vi "Shared Var Loop.vi"(0 "reference in":refnum<class "Stand.lvclass">, 11 "error in (no error)":errorcluster) -> (4 "reference in 2":refnum<class "Stand.lvclass">, 15 "error out":errorcluster)   [LabVIEW 2019, in "Stand.lvclass"]
uses:
  Stand.lvclass
  TypeDef/NVM Data.ctl
  modbus engine custom/MB_ENGINE_class/Engine Alarms.ctl
  modbus engine custom/MB_ENGINE_class/Engine State.ctl
  TypeDef/StateValveModbus.ctl
  modbus engine custom/MB_ENGINE_class/Settings.ctl
  Stand.lvclass/Stand.ctl
  ValveModbus_class/ValveModbus.lvclass/ValveModbus.ctl
  Engine_1DI_2DO_class/Engine_1DI_2DO.lvclass/Engine_1DI_2DO.ctl
  Sig_DA_class/Sig_DA.lvclass/Sig_DA.ctl
  TypeDef/DA_Data.ctl
  TypeDef/bool_data.ctl
  TypeDef/State HI_PERESS_TEST.ctl
  TypeDef/State.ctl
  Sig_AO_class/Sig_AO.lvclass/Sig_AO.ctl
  Sig_DO_Simple_class/Sig_DO_Simple.lvclass/Sig_DO_Simple.ctl
  Sig_DI_Simple_class/Sig_DI_Simple.lvclass/Sig_DI_Simple.ctl
  Sig_AI_class/Sig_AI.lvclass/Sig_AI.ctl
  AnalogComparator_class/AnalogComparator.lvclass/AnalogComparator.ctl
  TypeDef/AI_Data_Array.ctl
  TypeDef/AI_Data.ctl
  TypeDef/PumpData.ctl
  TypeDef/StatePump.ctl
  AnalogComparator_class/GetStatus.vi
  AnalogComparator_class/GetTh.vi
  modbus engine custom/MB_ENGINE_class/MB_ENGINE.lvclass
  Sig_AI_class/Sig_AI.lvclass
  Sig_DI_Simple_class/Sig_DI_Simple.lvclass
  Sig_DO_Simple_class/Sig_DO_Simple.lvclass
  Sig_AO_class/Sig_AO.lvclass
  Engine_1DI_2DO_class/Engine_1DI_2DO.lvclass
  Sig_DA_class/Sig_DA.lvclass
  ValveModbus_class/ValveModbus.lvclass
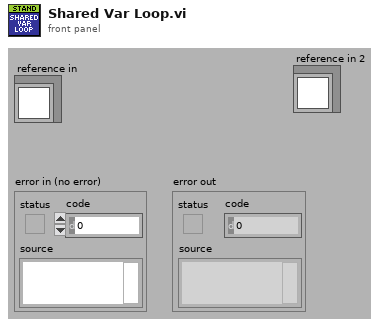
[diagram p1: front panel]
types:
  T1 = typedef "NVM Data.ctl" = cluster{"Alarms":T2, "Engine State":T3, "RAW Possition":i32, "StateValveModbus":T4, "Angele":dbl, "Step":i32, "Encoder":i32, "Kinematic":T5}
  T2 = typedef "MB_ENGINE.lvclass/Engine Alarms.ctl" = cluster{"OL":bool, "TF":bool, "STL":bool, "OCP":bool, "CPUV":bool, "UVLO":bool, "SPI_ERROR":bool, "Fault":bool, "OL 2":bool, "TF 2":bool, "STL 2":bool, "OCP 2":bool, "CPUV 2":bool, "UVLO 2":bool, "reserved":bool, "InitDone":bool}
  T3 = typedef "MB_ENGINE.lvclass/Engine State.ctl" = u16
  T4 = typedef "StateValveModbus.ctl" = enum16{"IDLE", "OPEN", "CLOSE", "OPENING", "CLOSING", "STOP"}
  T5 = typedef "MB_ENGINE.lvclass/Settings.ctl" = cluster{"ACC Steps Per Sec^2":u16, "DEC Steps Per Sec^2":u16, "Min Velosity Step Per Sec":u16, "Max Velosity Step Per Sec":u16, "MicroStep":u16}
  T6 = typedef "State.ctl" = enum16{"INIT", "IDLE", "CHANNEL_TESTING", "OIL_FILLING", "PREPARE_TO_HI_PRESS", "HI_PRESSURE", "ALARM", "HI PRESSURE TEST"}
  T7 = typedef "State HI_PERESS_TEST.ctl" = enum16{"NOT READY", "READY TO SUPPLY AIR", "PREPARE TO HI PRESS", "READY FOR HI PRESS", "CHECK DIRECTION", "INCREASING PRESSURE", "HOLDING", "PRESSURE RELEASE", "SOFT PRESSURE RELIEF", "ALARM"}
  T8 = typedef "StatePump.ctl" = enum16{"Off", "TupningOn", "On", "TurningOff"}
  T9 = typedef "AI_Data.ctl" = cluster{"Raw":dbl, "Scaled":dbl, "OutOfRangeMax":bool, "OutOfRangeMin":bool, "HIHI":bool, "HI":bool, "LO":bool, "LOLO":bool, "OutOfRangeMax_val":dbl, "OutOfRangeMin_val":dbl, "HIHI_val":dbl, "HI_val":dbl, "LO_val":dbl, "LOLO_val":dbl}
  T10 = typedef "bool_data.ctl" = cluster{"CURR":bool, "RAW_PREV":bool, "millisecond timer value":u32}
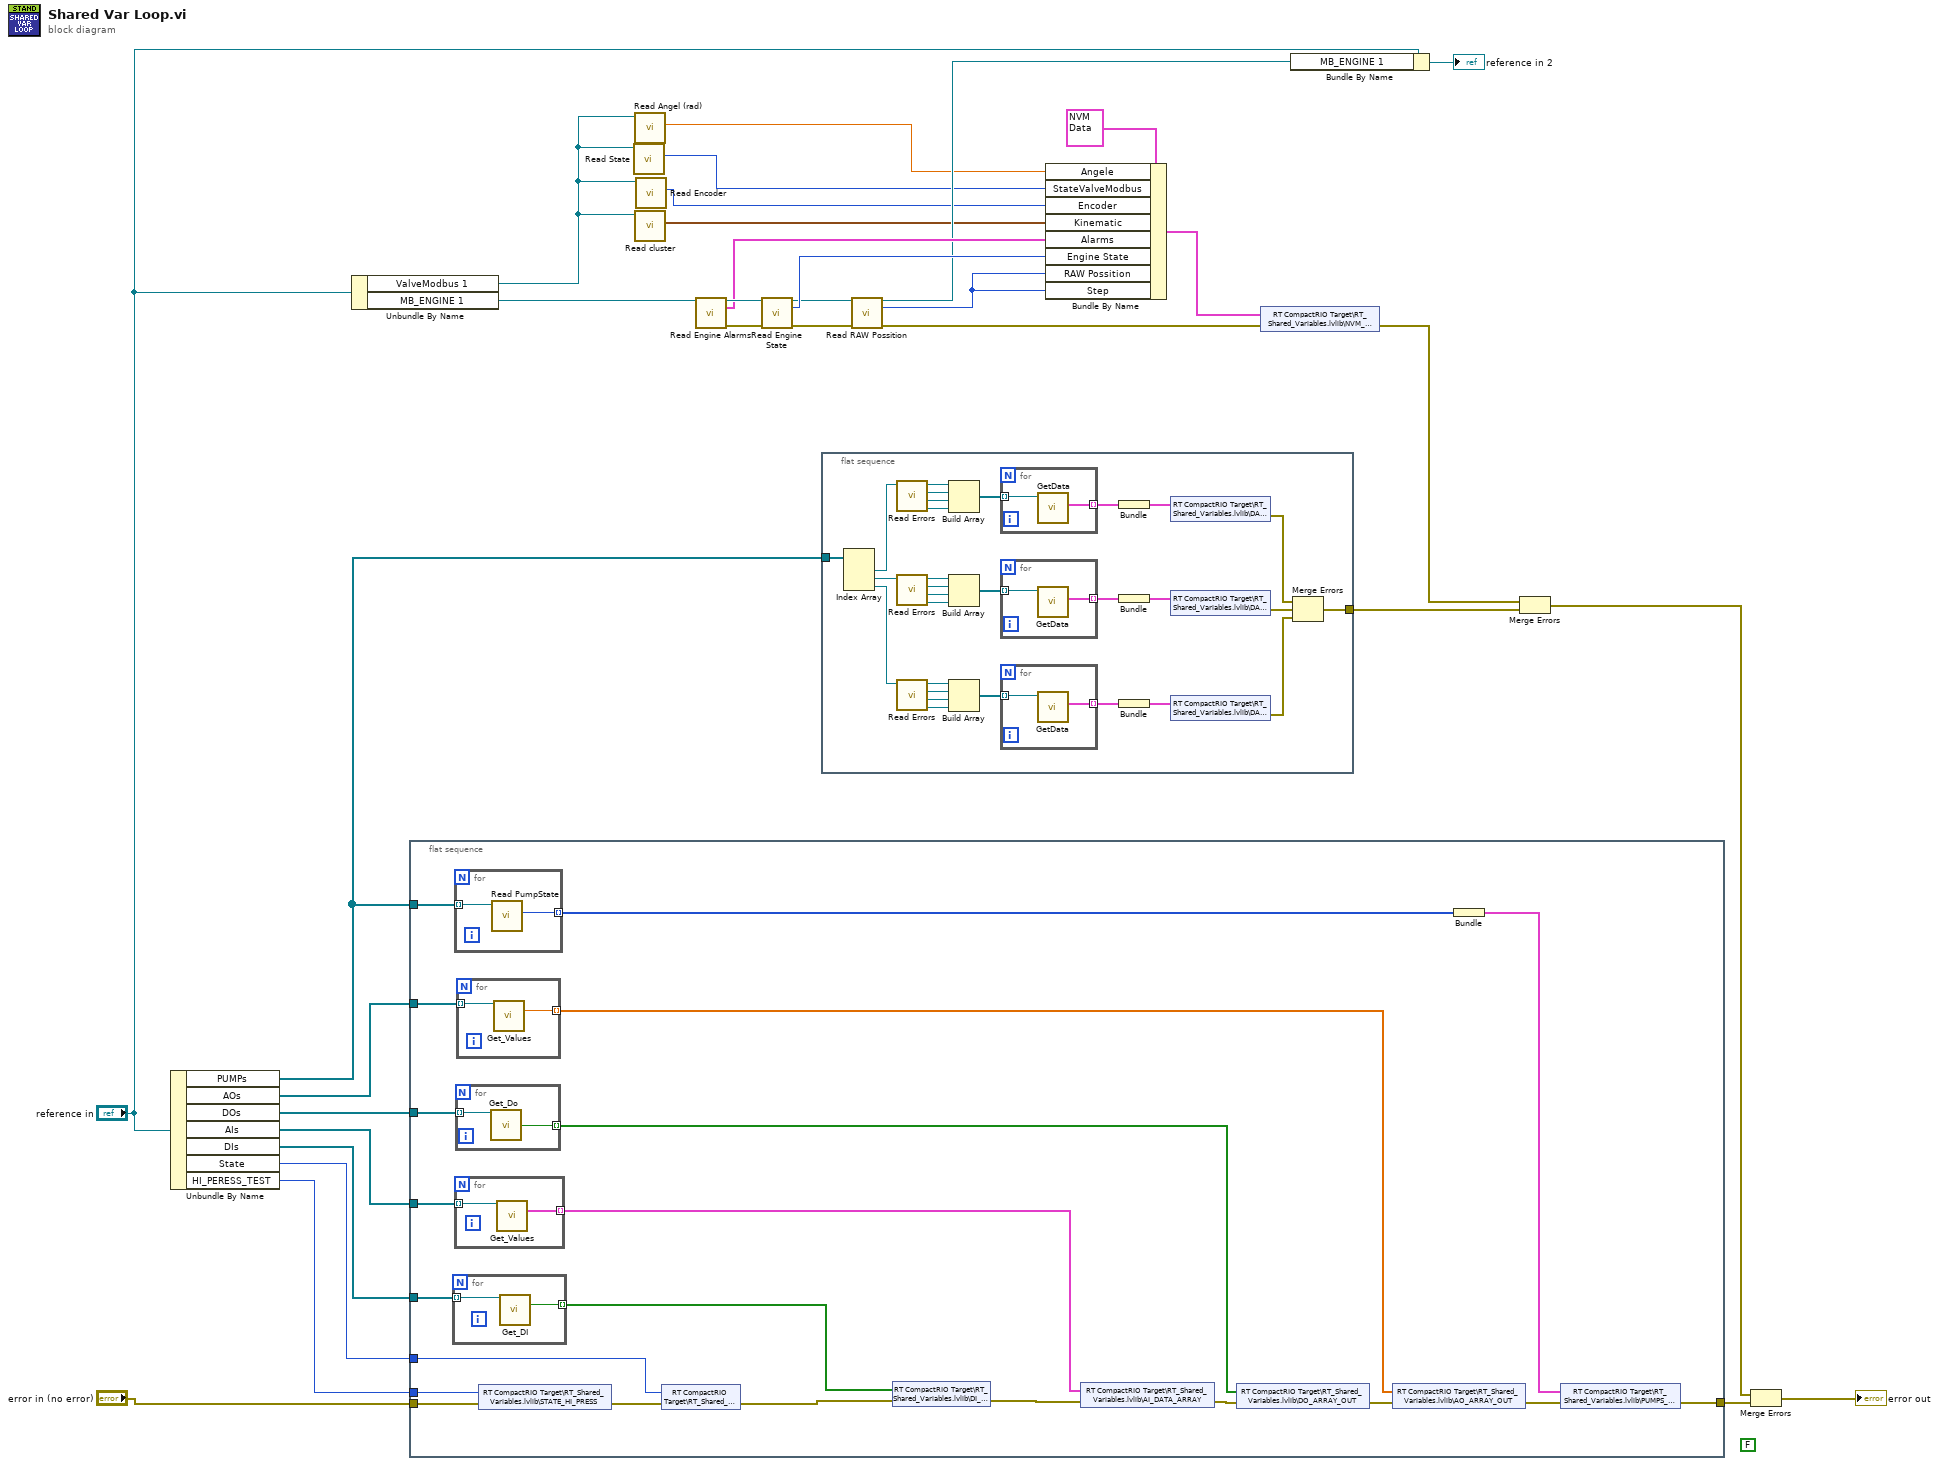
[diagram p0: block diagram]
diagram:
  (unwired) FALSE
  n1 = Unbundle By Name("reference in") -> ("PUMPs"=w27:refnum<class "Engine_1DI_2DO.lvclass">[], "AOs"=w28:refnum<class "Sig_AO.lvclass">[], "DOs"=w29:refnum<class "Sig_DO_Simple.lvclass">[], "AIs"=w31:refnum<class "Sig_AI.lvclass">[], "DIs"=w30:refnum<class "Sig_DI_Simple.lvclass">[], "State"=w23:T6, "HI_PERESS_TEST"=w1:T7)
  n2 = Unbundle By Name("reference in") -> ("ValveModbus 1"=w6:refnum<class "ValveModbus.lvclass">, "MB_ENGINE 1"=w14:refnum<class "MB_ENGINE.lvclass">)
  n3 = flat-sequence {
    tunnel: w31 -> [w53]
    tunnel: w30 -> [w51]
    tunnel: w29 -> [w49]
    tunnel: w28 -> [w47]
    tunnel: w27 -> [w41]
    tunnel: [w40] -> w26
    tunnel: "error in (no error)" -> [w34]
    tunnel: w23 -> [w39]
    tunnel: w1 -> [w35]
    frame #0 {
      n4 = for {
        tunnel: w51 -> [w61] mode=indexing
        tunnel: [w60] -> w38 mode=indexing
        n5 = call "Get_DI.vi"("reference in"=w61) -> ("DI"=w60:bool)  [unwired: 14 in]
      }
      n6 = for {
        tunnel: w41 -> [w55] mode=indexing
        tunnel: [w54] -> w43 mode=indexing
        n7 = call "Read PumpState.vi"("Pump_1AI_1DO_2DI in"=w55) -> ("PumpState"=w54:T8)  [unwired: 10 in]
      }
      n8 = for {
        tunnel: w53 -> [w63] mode=indexing
        tunnel: [w62] -> w52 mode=indexing
        n9 = call "Get_Values.vi"("reference in"=w63) -> ("Data"=w62:T9)  [unwired: 13 in, 1 out]
      }
      n10 = for {
        tunnel: w49 -> [w59] mode=indexing
        tunnel: [w58] -> w50 mode=indexing
        n11 = call "Get_Do.vi"("reference in"=w59) -> ("DO"=w58:bool)  [unwired: 14 in]
      }
      n12 = for {
        tunnel: w47 -> [w57] mode=indexing
        tunnel: [w56] -> w45 mode=indexing
        n13 = call "Get_Values.vi"("reference in"=w57) -> ("AO"=w56:dbl)  [unwired: 14 in]
      }
      n14 = shared-variable "RT CompactRIO Target\\RT_Shared_Variables.lvlib\\STATE_HI_PRESS"(w35, error in=w34) -> (error out=w33:errorcluster)
      n15 = shared-variable "RT CompactRIO Target\\RT_Shared_Variables.lvlib\\STATE"(w39, error in=w33) -> (error out=w37:errorcluster)
      n16 = shared-variable "RT CompactRIO Target\\RT_Shared_Variables.lvlib\\DI_ARRAY"(w38, error in=w37) -> (error out=w36:errorcluster)
      n17 = shared-variable "RT CompactRIO Target\\RT_Shared_Variables.lvlib\\AI_DATA_ARRAY"(w52, error in=w36) -> (error out=w48:errorcluster)
      n18 = shared-variable "RT CompactRIO Target\\RT_Shared_Variables.lvlib\\DO_ARRAY_OUT"(w50, error in=w48) -> (error out=w46:errorcluster)
      n19 = shared-variable "RT CompactRIO Target\\RT_Shared_Variables.lvlib\\AO_ARRAY_OUT"(w45, error in=w46) -> (error out=w44:errorcluster)
      n20 = Bundle(w43) -> (w42:cluster{T8[]})  [unwired: 1 in]
      n21 = shared-variable "RT CompactRIO Target\\RT_Shared_Variables.lvlib\\PUMPS_DATA"(w42, error in=w44) -> (error out=w40:errorcluster)
    }
  }
  n22 = call "Read State.vi"("Pump_1AI_1DO_2DI in"=w6) -> ("StateValveModbus"=w7:T4)  [unwired: 10 in]
  n23 = call "Read Angel (rad).vi"("ValveModbus in"=w6) -> ("Angel (rad)"=w5:dbl)  [unwired: 9 in, 1 out]
  n24 = call "Read cluster.vi"("ValveModbus in"=w6) -> ("cluster"=w8:T5)  [unwired: 9 in, 1 out]
  n25 = call "Read Encoder.vi"("ValveModbus in"=w6) -> ("Encoder"=w9:i32)  [unwired: 9 in, 1 out]
  n26 = call-dynamic "Read Engine Alarms.vi"("class data in"=w14) -> ("class data out"=w20:refnum<class "MB_ENGINE.lvclass">, "Alarms"=w18:T2, "error out"=w19:errorcluster)  [unwired: 12 in]
  n27 = call-dynamic "Read Engine State.vi"("class data in"=w20, "error in (no error)"=w19) -> ("class data out"=w16:refnum<class "MB_ENGINE.lvclass">, "Engine State"=w17:T3, "error out"=w15:errorcluster)  [unwired: 11 in]
  n28 = flat-sequence {
    tunnel: w27 -> [w92]
    tunnel: [w64] -> w25
    frame #0 {
      n29 = Index Array(array=w92) -> (element #1=w87:refnum<class "Engine_1DI_2DO.lvclass">, element #2=w82:refnum<class "Engine_1DI_2DO.lvclass">, element #3=w79:refnum<class "Engine_1DI_2DO.lvclass">)  [unwired: 3 in]
      n30 = call "Read Errors.vi"("Pump_1AI_1DO_2DI in"=w87) -> ("UnOFF Error"=w88:refnum<class "Sig_DA.lvclass">, "UnON Error"=w89:refnum<class "Sig_DA.lvclass">, "OFF Error"=w90:refnum<class "Sig_DA.lvclass">, "ON Error"=w91:refnum<class "Sig_DA.lvclass">)  [unwired: 7 in]
      n31 = call "Read Errors.vi"("Pump_1AI_1DO_2DI in"=w82) -> ("UnOFF Error"=w86:refnum<class "Sig_DA.lvclass">, "UnON Error"=w85:refnum<class "Sig_DA.lvclass">, "OFF Error"=w84:refnum<class "Sig_DA.lvclass">, "ON Error"=w83:refnum<class "Sig_DA.lvclass">)  [unwired: 7 in]
      n32 = call "Read Errors.vi"("Pump_1AI_1DO_2DI in"=w79) -> ("UnOFF Error"=w80:refnum<class "Sig_DA.lvclass">, "UnON Error"=w81:refnum<class "Sig_DA.lvclass">, "OFF Error"=w77:refnum<class "Sig_DA.lvclass">, "ON Error"=w78:refnum<class "Sig_DA.lvclass">)  [unwired: 7 in]
      n33 = Build Array(w91, w90, w89, w88) -> (w76:refnum<class "Sig_DA.lvclass">[])
      n34 = Build Array(w83, w84, w85, w86) -> (w72:refnum<class "Sig_DA.lvclass">[])
      n35 = Build Array(w78, w77, w81, w80) -> (w71:refnum<class "Sig_DA.lvclass">[])
      n36 = for {
        tunnel: w76 -> [w98] mode=indexing
        tunnel: [w97] -> w74 mode=indexing
        n37 = call "GetData.vi"("Sig_DA in"=w98) -> ("data"=w97:T10)  [unwired: 10 in]
      }
      n38 = for {
        tunnel: [w96] -> w73 mode=indexing
        tunnel: w72 -> [w95] mode=indexing
        n39 = call "GetData.vi"("Sig_DA in"=w95) -> ("data"=w96:T10)  [unwired: 10 in]
      }
      n40 = for {
        tunnel: [w94] -> w70 mode=indexing
        tunnel: w71 -> [w93] mode=indexing
        n41 = call "GetData.vi"("Sig_DA in"=w93) -> ("data"=w94:T10)  [unwired: 10 in]
      }
      n42 = Bundle(w74) -> (w75:cluster{T10[]})  [unwired: 1 in]
      n43 = Bundle(w73) -> (w68:cluster{T10[]})  [unwired: 1 in]
      n44 = Bundle(w70) -> (w69:cluster{T10[]})  [unwired: 1 in]
      n45 = shared-variable "RT CompactRIO Target\\RT_Shared_Variables.lvlib\\DA_ENG_0"(w75) -> (error out=w65:errorcluster)  [unwired: 1 in]
      n46 = shared-variable "RT CompactRIO Target\\RT_Shared_Variables.lvlib\\DA_ENG_1"(w68) -> (error out=w66:errorcluster)  [unwired: 1 in]
      n47 = shared-variable "RT CompactRIO Target\\RT_Shared_Variables.lvlib\\DA_ENG_2"(w69) -> (error out=w67:errorcluster)  [unwired: 1 in]
      n48 = Merge Errors(w65, w66, w67) -> (w64:errorcluster)
    }
  }
  n49 = call-dynamic "Read RAW Possition.vi"("class data in"=w16, "error in (no error)"=w15) -> ("class data out"=w11:refnum<class "MB_ENGINE.lvclass">, "RAW Possition"=w10:i32, "error out"=w4:errorcluster)  [unwired: 11 in]
  n50 = Bundle By Name(cluster=T1 {"Alarms"={"OL"=FALSE, "TF"=FALSE, "STL"=FALSE, "OCP"=FALSE, "CPUV"=FALSE, "UVLO"=FALSE, "SPI_ERROR"=FALSE, "Fault"=FALSE, "OL 2"=FALSE, "TF 2"=FALSE, "STL 2"=FALSE, "OCP 2"=FALSE, "CPUV 2"=FALSE, "UVLO 2"=FALSE, "reserved"=TRUE, "InitDone"=TRUE}, "Engine State"=8, "RAW Possition"=124110, "StateValveModbus"=enum."IDLE", "Angele"=0.0, "Step"=0, "Encoder"=0, "Kinematic"={"ACC Steps Per Sec^2"=100, "DEC Steps Per Sec^2"=100, "Min Velosity Step Per Sec"=100, "Max Velosity Step Per Sec"=200, "MicroStep"=16}} ("NVM_DATA_1"), "Angele"=w5, "StateValveModbus"=w7, "Encoder"=w9, "Kinematic"=w8, "Alarms"=w18, "Engine State"=w17, "RAW Possition"=w10, "Step"=w10) -> (w21:T1)
  n51 = shared-variable "RT CompactRIO Target\\RT_Shared_Variables.lvlib\\NVM_DATA_1"(w21, error in=w4) -> (error out=w2:errorcluster)
  n52 = Bundle By Name(cluster="reference in", "MB_ENGINE 1"=w11) -> (→"reference in 2":refnum<class "Stand.lvclass">)
  n53 = Merge Errors(w2, w25) -> (w3:errorcluster)
  n54 = Merge Errors(w3, w26) -> (→"error out":errorcluster)
